vi "FileMan Print File.vi"(8 "error in (no error)":errorcluster, 9 "show (1:Normal)":i16(ring)=1 items=["SW_HIDE", "SW_SHOWNORMAL", "SW_SHOWMINIMIZED"], 10 "path to file (empty path)":path) -> (0 "error out":errorcluster)   [LabVIEW 2023, in "Winevent.lvlib"]
doc: "This VI will print a file whose extension is associated with an application, as available in Windows' File Manager. For example, files with the .wri extension are usually associated with the Windows application Write. A file with the extension .wri will then be printed using Microsoft Write.\n\nFiles whose extensions are not associated with an application, or applications which do not support file printing from the File Manager, will return an error."
uses:
  Winevent.lvlib
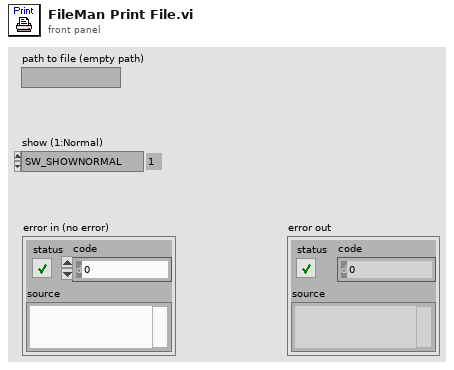
[diagram p1: front panel]
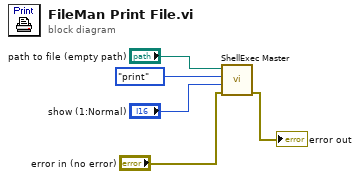
[diagram p0: block diagram]
diagram:
  n1 = call "ShellExec Master.vi"("error in (no error)"="error in (no error)", "show"="show (1:Normal)", "operation"=enum16{"open", "print"}."print", "path to file"="path to file (empty path)") -> ("error out"=→"error out":errorcluster)  [unwired: 2 in, 3 out]
